vi "Flip Tile Vertical.vi"(8 "error in (no error)":errorcluster, 11 "Tile in":refnum<class "Tile.lvclass">) -> (0 "error out":errorcluster, 3 "Tile out":refnum<class "Tile.lvclass">)   [LabVIEW 2020, in "Tile.lvclass"]
uses:
  Tile.lvclass
  Tile.lvclass/Tile.ctl
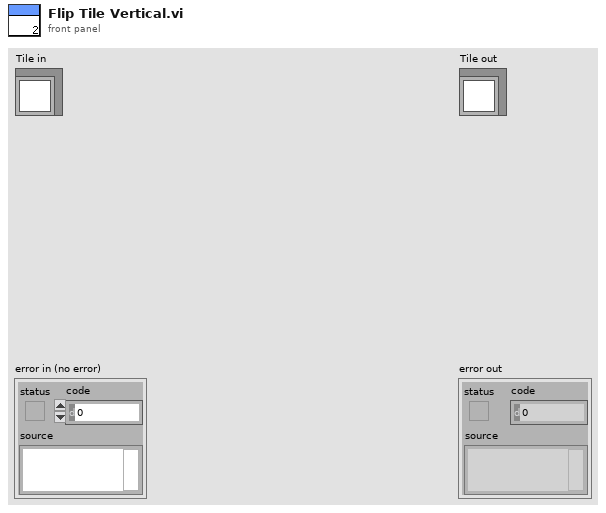
[diagram p1: front panel]
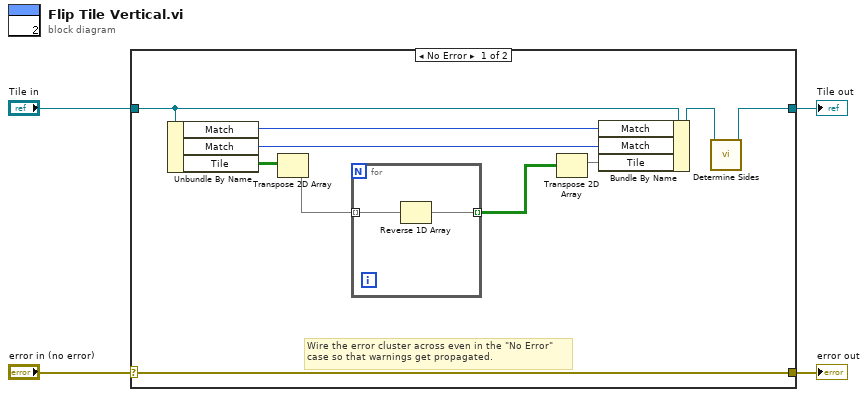
[diagram p0: block diagram]
diagram:
  n1 = case shown="No Error" "error in (no error)" {
    selector: "error in (no error)" -> [w14 w18]
    tunnel: [w14 w18] -> w3
    tunnel: [w9 w17] -> w1
    tunnel: "Tile in" -> [w11 w17]
    frame No Error {
      # "Wire the error cluster across even in the \"No Error\"\ncase so that warnings get propagated."
      n2 = Unbundle By Name(w11) -> ("Match"=w7:u64, "Match"=w8:u64, "Tile"=w13:bool[][])
      n3 = Transpose 2D Array(2D array=w13) -> (transposed array=w6:bool[][])
      n4 = for {
        tunnel: w6 -> [w16] mode=indexing
        tunnel: [w15] -> w5 mode=indexing
        n5 = Reverse 1D Array(array=w16) -> (reversed array=w15:bool[])
      }
      n6 = Transpose 2D Array(2D array=w5) -> (transposed array=w12:bool[][])
      n7 = Bundle By Name(cluster=w11, "Match"=w7, "Match"=w8, "Tile"=w12) -> (w10:refnum<class "Tile.lvclass">)
      n8 = call "Determine Sides.vi"("Tile in"=w10) -> ("Tile out"=w9:refnum<class "Tile.lvclass">)  [unwired: 9 in, 1 out]
    }
    frame Error {
    }
  }
  "error out" <- w3
  "Tile out" <- w1
